vi "Set Strings[4].vi"(9 "index (row)":i32, 10 "Array":string[][](array[string]), 11 "Control in":refnum<vi>) -> (0 "error out":errorcluster, 3 "Control out":refnum<vi>)   [LabVIEW 2016]
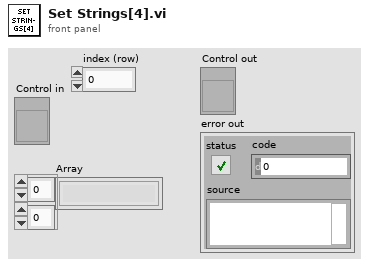
[diagram p1: front panel]
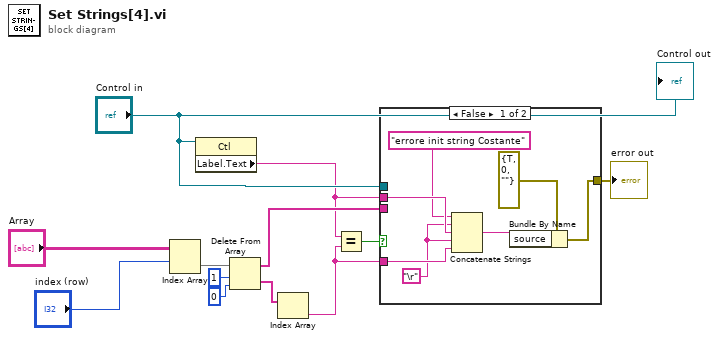
[diagram p0: block diagram]
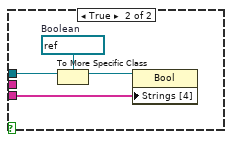
[diagram p2: hidden frame]
diagram:
  n1 = Index Array(array="Array", index (row)="index (row)") -> (element=w9:string[])  [unwired: 1 in]
  n2 = property class="Ctl"(reference="Control in") -> ("Label.Text"=w2:string)  [unwired: 1 in, 2 out]
  n3 = Delete From Array(array=w9, length=1, index=0) -> (deleted portion=w6:string[], array with subset deleted=w12:string[])
  n4 = Index Array(array=w6) -> (element=w1:string)  [unwired: 1 in]
  n5 = Equal?(x=w2, y=w1) -> (x = y?=w5:bool)
  n6 = case shown="False" w5 {
    tunnel: w12 -> [_ w23]
    tunnel: "Control in" -> [_ w20]
    tunnel: [w18 _] -> w3
    tunnel: w2 -> [w16 _]
    tunnel: w1 -> [w15 _]
    frame False {
      w14 = "\r"
      n7 = Concatenate Strings("errore init string Costante" ("string"), w14, w16, w14, w15) -> (w17:string)
      n8 = Bundle By Name(cluster=errorcluster {"status"=TRUE, "code"=0, "source"=""} ("error out"), "source"=w17) -> (w18:errorcluster)
    }
    frame True {
      w21 = refnum<vi> refnum  # Boolean
      n9 = To More Specific Class(target class=w21, reference=w20) -> (specific class reference=w22:refnum<vi>)  [unwired: 1 in, 1 out]
      n10 = property class="Bool"(reference=w22, "Strings [4]"=w23) -> ()  [unwired: 1 in, 2 out]
    }
  }
  "error out" <- w3
  "Control out" <- "Control in"
